vi "Test CE14_v2 API.vi"() -> ()   [LabVIEW 2018]
doc: "CE14_v2 API Tester."
uses:
  Instrument Drivers/LVdriver_CE14(eMIC)/type defs/CE14.data.ctl
  CE14_v2.lvlib
  Instrument Drivers/LVdriver_CE14(eMIC)/CE14_eMIC.lvlib
panel:
  in  "Connect to CE14":bool
  out "Array":T1[](array[typedef])
  in  "CE14_response":bool
  in  "Read AC parameters":bool
  out "Success?":bool
  in  "CE14.ShakeHand":bool
  in  "VISA resource name":refnum<visa-resource-name>
  in  "Run as Singleton?":bool
  in  "Show Block Diagram":bool
  in  "Refresh Modules":bool
  out "Active Modules":string[](array[string])
  in  "Stop Module":bool
  in  "Select Module":i32(ring)=-1 caption="Select Module\nTo send Request to" items=["All"=-1, "1"=1]
  in  "Run New Module":bool
  in  "Hide Module Panel":bool
  in  "Show Module Panel":bool
  out "Status":string
  # "This VI tests the API for the Module."
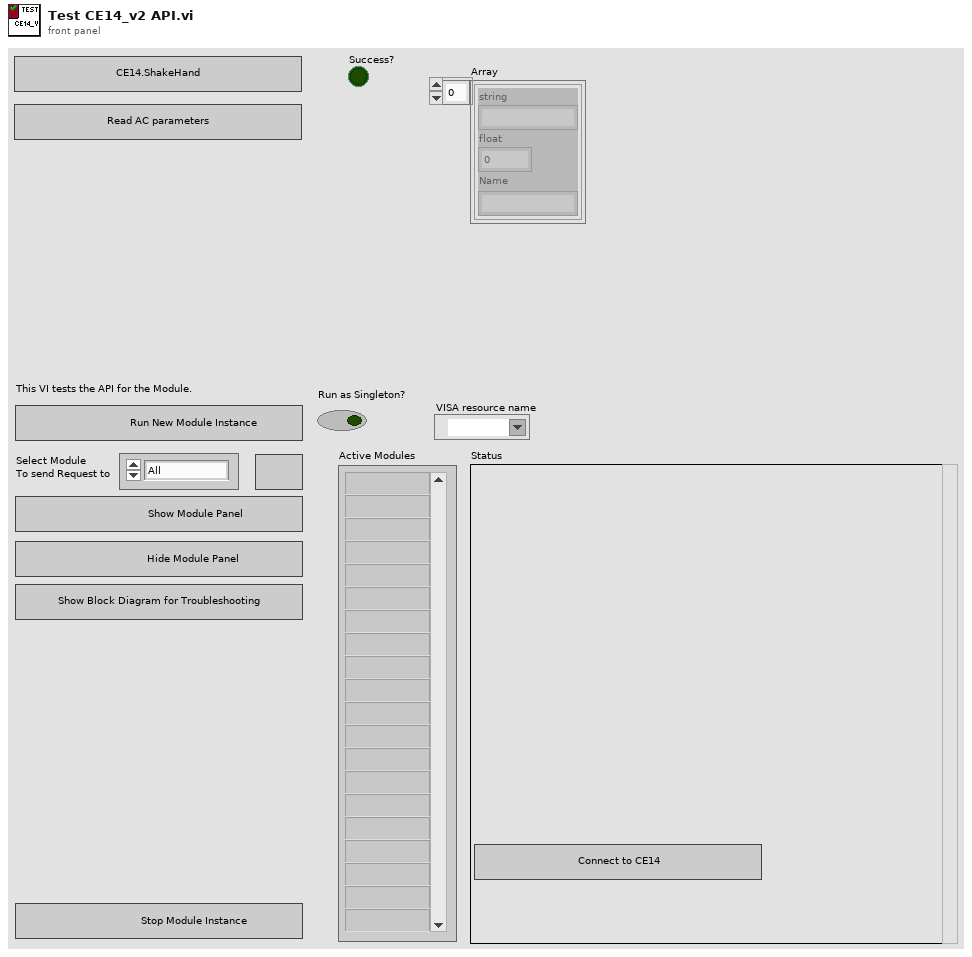
[diagram p1: front panel]
types:
  T1 = typedef "CE14_eMIC.lvlib/CE14.data.ctl" = cluster{"string":string, "float":dbl, "Name":string}
  T2 = typedef "CE14_v2.lvlib/Broadcast Events--cluster.ctl" = cluster{"Module Did Init":refnum<user-event>, "Status Updated":refnum<user-event>, "Error Reported":refnum<user-event>, "Module Did Stop":refnum<user-event>, "Update Module Execution Status":refnum<user-event>, "CE14 response data":refnum<user-event>}
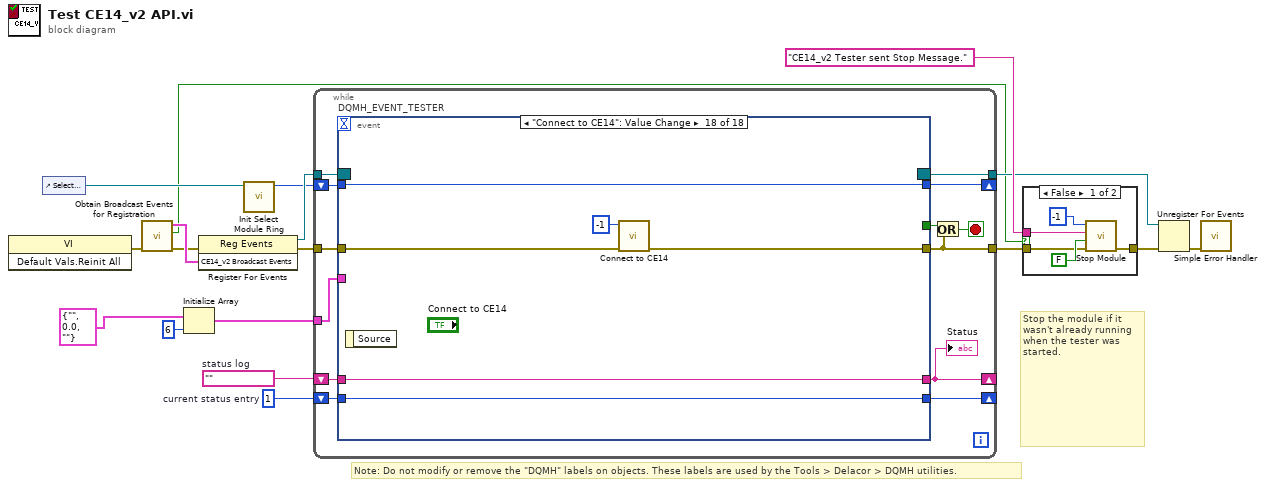
[diagram p0: block diagram]
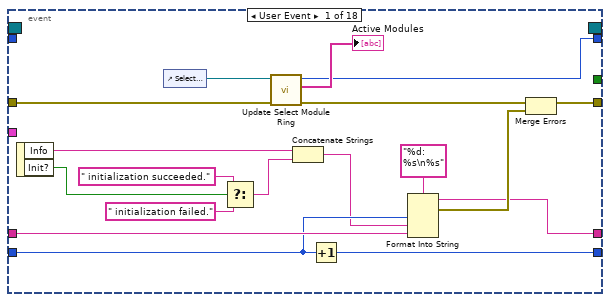
[diagram p3: hidden frame]
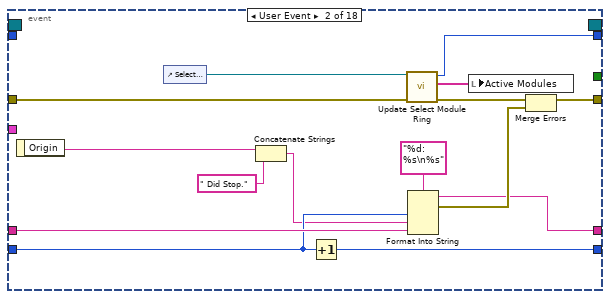
[diagram p4: hidden frame]
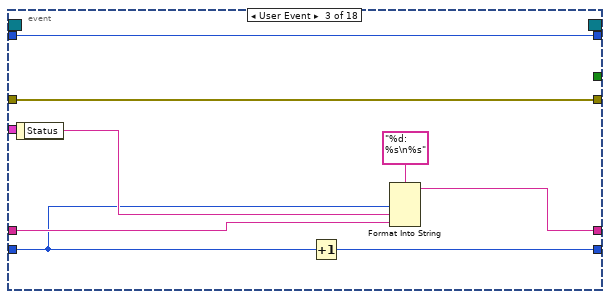
[diagram p5: hidden frame]
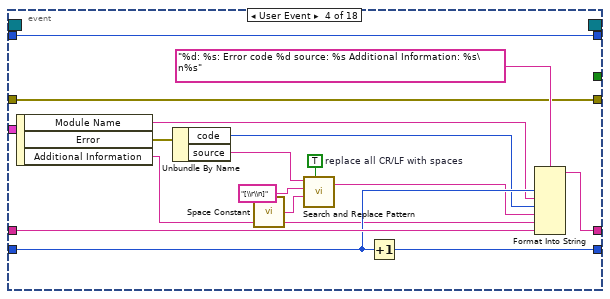
[diagram p6: hidden frame]
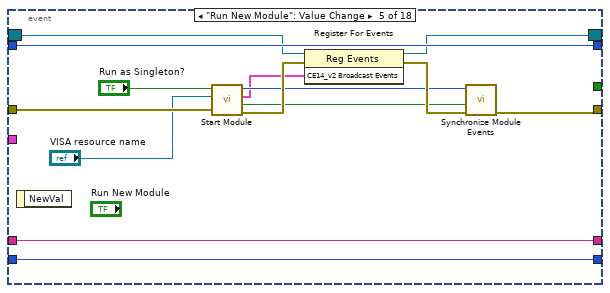
[diagram p7: hidden frame]
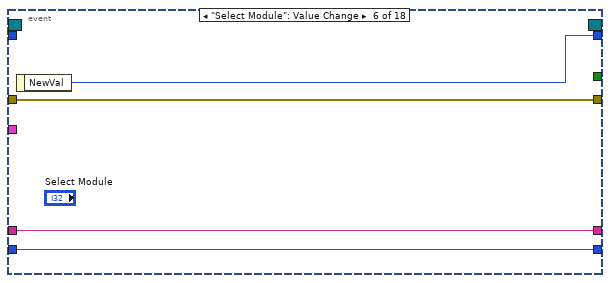
[diagram p8: hidden frame]
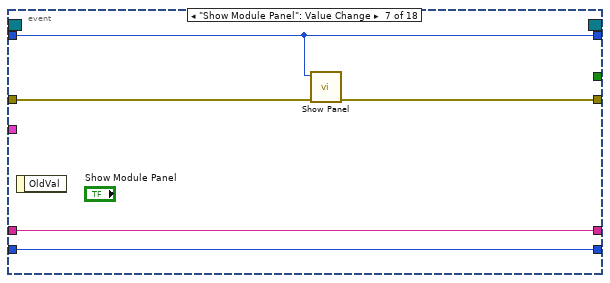
[diagram p9: hidden frame]
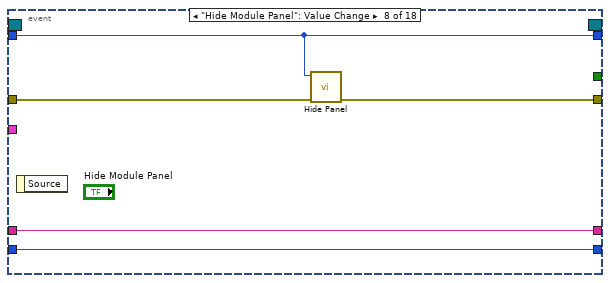
[diagram p10: hidden frame]
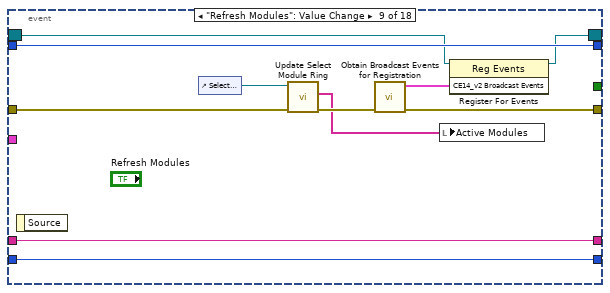
[diagram p11: hidden frame]
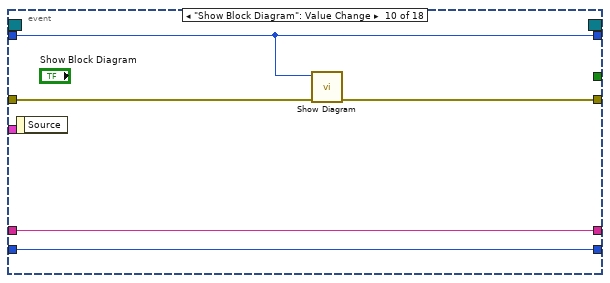
[diagram p12: hidden frame]
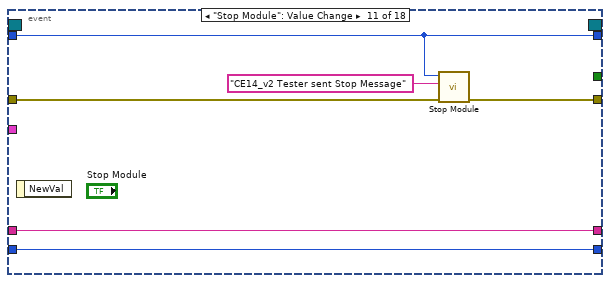
[diagram p13: hidden frame]
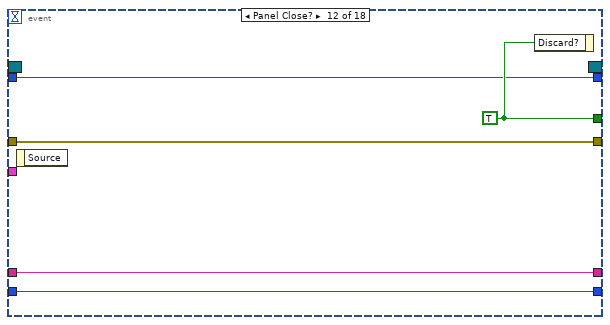
[diagram p14: hidden frame]
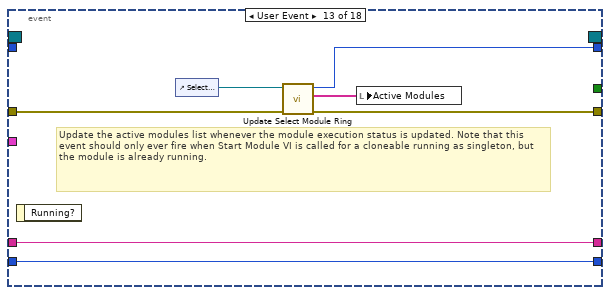
[diagram p15: hidden frame]
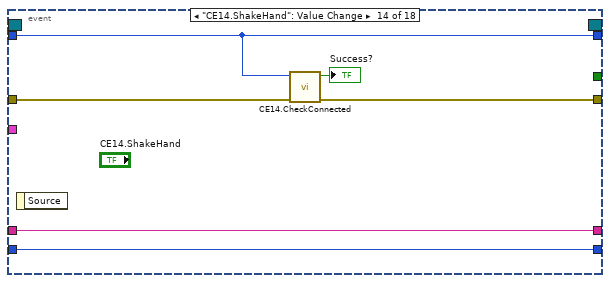
[diagram p16: hidden frame]
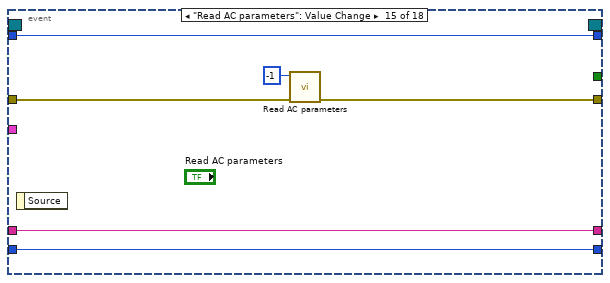
[diagram p17: hidden frame]
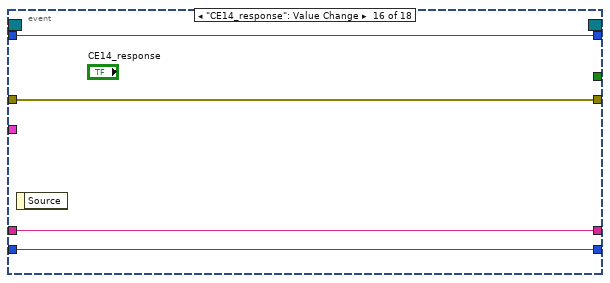
[diagram p18: hidden frame]
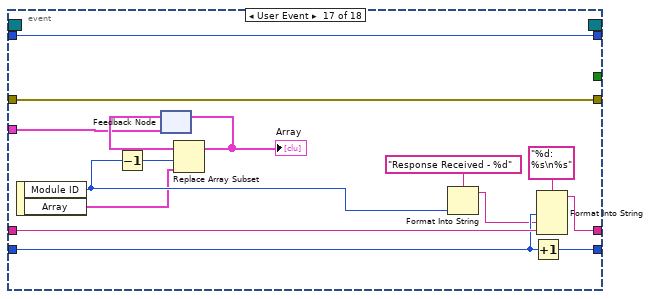
[diagram p19: hidden frame]
diagram:
  w15 = 1  # current status entry
  w16 = ""  # status log
  # "Stop the module if it wasn't already running when the tester was started."
  # "Note: Do not modify or remove the \"DQMH\" labels on objects. These labels are used by the Tools > Delacor > DQMH utilities."
  n1 = invoke class="VI" method="Default Vals.Reinit All"() -> (error out=w8:errorcluster)  [unwired: 3 in, 2 out]
  n2 = control-ref of="Select Module"() -> (w13:refnum<vi>)
  n3 = call "Obtain Broadcast Events for Registration.vi"("error in (no error)"=w8) -> ("error out"=w7:errorcluster, "Already running?"=w6:bool, "CE14_v2 Broadcast Events"=w12:T2)  [unwired: 8 in]
  n4 = Initialize Array(T1 {"string"="", "float"=0.0, "Name"=""} ("CE14. Data"), 6 ("dimension size")) -> (w1:T1[])
  n5 = register-events(error in=w7, w12) -> (reference out=w18:refnum<event-registration>, error out=w11:errorcluster)  [unwired: 1 in]
  n6 = call "Init Select Module Ring.vi"("Select Module Ring Ref"=w13) -> ("Value for All Modules"=w14:i32)  [unwired: 8 in, 2 out]
  n7 = while {
    tunnel: w18 -> [w31]
    tunnel: [w20] -> w5
    tunnel: w11 -> [w29]
    shift-right: [w25] -> _
    shift-left: w16 -> [w27]
    shift-right: [w26] -> _
    shift-left: w15 -> [w28]
    shift-right: [w22] -> _
    shift-left: w14 -> [w23]
    tunnel: [w21] -> w9
    tunnel: w1 -> [w19]
    stop <- w24 stop-if-true
    n8 = event "DQMH_EVENT_TESTER" shown="[17] \"Connect to CE14\": Value Change" {
      selector: w31 -> [_ _ _ _ w96 _ _ _ w122 _ _ _ _ _ _ _ _ _]
      dyn-events: [_ _ _ _ w95 _ _ _ w121 _ _ _ _ _ _ _ _ _] -> w21
      timeout: _ -> [_ _ _ _ _ _ _ _ _ _ _ _ _ _ _ _ _ _]
      tunnel: [_ _ _ _ _ _ _ _ _ _ _ w143 _ _ _ _ _ _] -> w30
      tunnel: [w39 w56 w72 w78 w94 w106 w110 w115 w118 w129 w134 w142 w146 w153 w158 w163 w181 w183] -> w20
      tunnel: w29 -> [w41 w58 w72 w78 w97 w106 w111 w116 w123 w132 w135 w142 w147 w156 w162 w163 w181 w187]
      tunnel: w28 -> [w46 w61 w65 w84 w99 w104 w108 w113 w126 w130 w137 w140 w149 w154 w160 w165 w177 w185]
      tunnel: w27 -> [w47 w62 w68 w86 w100 w105 w109 w114 w127 w131 w138 w141 w150 w155 w161 w166 w179 w186]
      tunnel: [w44 w59 w69 w81 w100 w105 w109 w114 w127 w131 w138 w141 w150 w155 w161 w166 w178 w186] -> w25
      tunnel: [w45 w60 w71 w87 w99 w104 w108 w113 w126 w130 w137 w140 w149 w154 w160 w165 w176 w185] -> w26
      tunnel: w23 -> [_ _ w66 w88 w98 _ w107 w112 w125 w128 w136 w139 _ w151 w159 w164 w180 w184]
      tunnel: [w36 w53 w66 w88 w98 w103 w107 w112 w125 w128 w136 w139 w145 w151 w159 w164 w180 w184] -> w22
      tunnel: w19 -> [_ _ _ _ _ _ _ _ _ _ _ _ _ _ _ _ w170 _]
      event User Event {
        n9 = event-data() -> ("Info"=w43:string, "Init?"=w33:bool)  [unwired: 1 in]
        n10 = control-ref of="Select Module"() -> (w38:refnum<vi>)
        n11 = Select(t=" initialization succeeded.", s=w33, f=" initialization failed.") -> (s? t:f=w32:string)
        n12 = call "Update Select Module Ring.vi"("error in (no error)"=w41, "Select Module Ring Ref"=w38) -> ("error out"=w40:errorcluster, "Active Modules (Array)"=→"Active Modules":string[], "New Module Ring Value"=w36:i32)  [unwired: 7 in]
        n13 = Concatenate Strings(w43, w32) -> (w42:string)
        n14 = Increment(x=w46) -> (x+1=w45:i32)
        n15 = Format Into String(format string="%d: %s\n%s", w46, w42, w47) -> (resulting string=w44:string, error out=w49:errorcluster)  [unwired: 2 in]
        n16 = Merge Errors(w40, w49) -> (w39:errorcluster)
      }
      event User Event {
        n17 = event-data() -> ("Origin"=w51:string)  [unwired: 1 in]
        n18 = control-ref of="Select Module"() -> (w55:refnum<vi>)
        n19 = Concatenate Strings(w51, " Did Stop.") -> (w50:string)
        n20 = Increment(x=w61) -> (x+1=w60:i32)
        n21 = call "Update Select Module Ring.vi"("error in (no error)"=w58, "Select Module Ring Ref"=w55) -> ("error out"=w57:errorcluster, "Active Modules (Array)"=w54:string[], "New Module Ring Value"=w53:i32)  [unwired: 7 in]
        n22 = Format Into String(format string="%d: %s\n%s", w61, w50, w62) -> (resulting string=w59:string, error out=w64:errorcluster)  [unwired: 2 in]
        n23 = local write "Active Modules"(w54) -> ()
        n24 = Merge Errors(w57, w64) -> (w56:errorcluster)
      }
      event User Event {
        n25 = event-data() -> ("Status"=w67:string)  [unwired: 1 in]
        n26 = Increment(x=w65) -> (x+1=w71:i32)
        n27 = Format Into String(format string="%d: %s\n%s", w65, w67, w68) -> (resulting string=w69:string)  [unwired: 2 in, 1 out]
      }
      event User Event {
        w82 = TRUE  # replace all CR/LF with spaces
        n28 = event-data() -> ("Module Name"=w76:string, "Error"=w75:errorcluster, "Additional Information"=w73:string)  [unwired: 1 in]
        n29 = Unbundle By Name(w75) -> ("code"=w77:i32, "source"=w79:string)
        n30 = call <vilib>:"Space Constant.vi"() -> ("String"=w83:string)
        n31 = call <vilib>:"Search and Replace Pattern.vi"("string"=w79, "regular expression (\"\")"="[\\r\\n]" ("regular expression (\"\")"), "replace string (\"\")"=w83, "replace all? (F)"=w82) -> ("result string"=w80:string)  [unwired: 1 in, 1 out]
        n32 = Increment(x=w84) -> (x+1=w87:i32)
        n33 = Format Into String(format string="%d: %s: Error code %d source: %s Additional Information: %s\n%s", w84, w76, w77, w80, w73, w86) -> (resulting string=w81:string)  [unwired: 2 in, 1 out]
      }
      event "Run New Module": Value Change {
        n34 = event-data() -> ()  [unwired: 1 in, 1 out]
        n35 = call "Start Module.vi"("error in"=w97, "VISA resource name"="VISA resource name", "Run as Singleton? (F)"="Run as Singleton?") -> ("error out"=w101:errorcluster, "Wait for Event Sync?"=w92:bool, "CE14_v2 Broadcast Events"=w91:T2, "Module ID"=w93:i32)  [unwired: 5 in]
        n36 = register-events(reference=w96, error in=w101, w91) -> (reference out=w95:refnum<event-registration>, error out=w102:errorcluster)
        n37 = call "Synchronize Module Events.vi"("error in"=w102, "Wait for Event Sync?"=w92, "Module ID in"=w93) -> ("error out"=w94:errorcluster)  [unwired: 7 in, 1 out]
      }
      event "Select Module": Value Change {
        n38 = event-data() -> ("NewVal"=w103:i32)  [unwired: 1 in]
      }
      event "Show Module Panel": Value Change {
        n39 = event-data() -> ()  [unwired: 1 in, 1 out]
        n40 = call "Show Panel.vi"("error in (no error)"=w111, "Module ID"=w107) -> ("error out"=w110:errorcluster)  [unwired: 9 in]
      }
      event "Hide Module Panel": Value Change {
        n41 = event-data() -> ()  [unwired: 1 in, 1 out]
        n42 = call "Hide Panel.vi"("error in (no error)"=w116, "Module ID"=w112) -> ("error out"=w115:errorcluster)  [unwired: 9 in]
      }
      event "Refresh Modules": Value Change {
        n43 = event-data() -> ()  [unwired: 1 in, 1 out]
        n44 = control-ref of="Select Module"() -> (w124:refnum<vi>)
        n45 = call "Update Select Module Ring.vi"("error in (no error)"=w123, "Select Module Ring Ref"=w124) -> ("error out"=w119:errorcluster, "Active Modules (Array)"=w117:string[])  [unwired: 7 in, 1 out]
        n46 = call "Obtain Broadcast Events for Registration.vi"("error in (no error)"=w119) -> ("error out"=w118:errorcluster, "CE14_v2 Broadcast Events"=w120:T2)  [unwired: 8 in, 1 out]
        n47 = local write "Active Modules"(w117) -> ()
        n48 = register-events(reference=w122, w120) -> (reference out=w121:refnum<event-registration>)  [unwired: 1 in, 1 out]
      }
      event "Show Block Diagram": Value Change {
        n49 = event-data() -> ()  [unwired: 1 in, 1 out]
        n50 = call "Show Diagram.vi"("error in (no error)"=w132, "Module ID"=w128) -> ("error out"=w129:errorcluster)  [unwired: 9 in]
      }
      event "Stop Module": Value Change {
        n51 = event-data() -> ()  [unwired: 1 in, 1 out]
        n52 = call "Stop Module.vi"("error in (no error)"=w135, "Origin"="CE14_v2 Tester sent Stop Message", "Module ID"=w136) -> ("error out"=w134:errorcluster)  [unwired: 8 in]
      }
      event Panel Close? {
        w143 = TRUE ("Discard?")
        n53 = event-data() -> ()  [unwired: 1 in, 1 out]
        n54 = event-data("Discard?"=w143) -> ()  [unwired: 1 in, 1 out]
      }
      event User Event {
        # "Update the active modules list whenever the module execution status is updated. Note that this event should only ever fire when Start Module VI is called for a cloneable running as singleton, but the module is already running."
        n55 = event-data() -> ()  [unwired: 1 in, 1 out]
        n56 = control-ref of="Select Module"() -> (w148:refnum<vi>)
        n57 = call "Update Select Module Ring.vi"("error in (no error)"=w147, "Select Module Ring Ref"=w148) -> ("error out"=w146:errorcluster, "Active Modules (Array)"=w144:string[], "New Module Ring Value"=w145:i32)  [unwired: 7 in]
        n58 = local write "Active Modules"(w144) -> ()
      }
      event "CE14.ShakeHand": Value Change {
        n59 = event-data() -> ()  [unwired: 1 in, 1 out]
        n60 = call "CE14.CheckConnected.vi"("error in"=w156, "Module ID"=w151) -> ("error out"=w153:errorcluster, "Success"=→"Success?":bool)  [unwired: 7 in, 1 out]
      }
      event "Read AC parameters": Value Change {
        n61 = event-data() -> ()  [unwired: 1 in, 1 out]
        n62 = call "Read AC parameters.vi"("error in"=w162, "Module ID"=-1) -> ("error out"=w158:errorcluster)  [unwired: 9 in]
      }
      event "CE14_response": Value Change {
        n63 = event-data() -> ()  [unwired: 1 in, 1 out]
      }
      event User Event {
        n64 = event-data() -> ("Module ID"=w172:i32, "Array"=w168:T1[])  [unwired: 1 in]
        n65 = Decrement(x=w172) -> (x-1=w169:i32)
        n66 = feedback #1(w170) -> (w171:T1[])
        n67 = Replace Array Subset(array=w171, new element=w168, index=w169) -> (w167:T1[])
        "Array" <- w167
        n68 = feedback-in #1(w167) -> ()
        n69 = Format Into String(format string="Response Received - %d", w172) -> (resulting string=w173:string)  [unwired: 2 in, 1 out]
        n70 = Increment(x=w177) -> (x+1=w176:i32)
        n71 = Format Into String(format string="%d: %s\n%s", w177, w173, w179) -> (resulting string=w178:string)  [unwired: 2 in, 1 out]
      }
      event "Connect to CE14": Value Change {
        n72 = event-data() -> ()  [unwired: 1 in, 1 out]
        n73 = call "Connect to CE14.vi"("error in"=w187, "Module ID"=-1) -> ("error out"=w183:errorcluster)  [unwired: 9 in]
      }
    }
    "Status" <- w25
    n74 = Or(x=w30, y=w20) -> (x .or. y?=w24:bool)
  }
  n75 = case shown="False" w6 {
    tunnel: [w192 w193] -> w17
    tunnel: "CE14_v2 Tester sent Stop Message." ("Origin") -> [w191 _]
    tunnel: w5 -> [w188 w193]
    frame False {
      n76 = call "Stop Module.vi"("error in (no error)"=w188, "Wait for Module to stop? (F)"=FALSE ("Wait for Module to stop?"), "Origin"=w191, "Module ID"=-1 ("Stop all")) -> ("error out"=w192:errorcluster)  [unwired: 7 in]
    }
    frame True {
    }
  }
  n77 = Unregister For Events(event registration refnum=w9, error in=w17) -> (error out=w4:errorcluster)
  n78 = call <vilib>:"Simple Error Handler.vi"("error in (no error)"=w4) -> ()  [unwired: 4 in, 5 out]
